vi "Was_string_matched.vi"(0 "Match Error":bool=TRUE, 1 "String Name":string, 2 "Variable name":string) -> ()   [LabVIEW 2010]
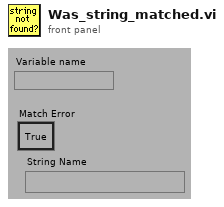
[diagram p1: front panel]
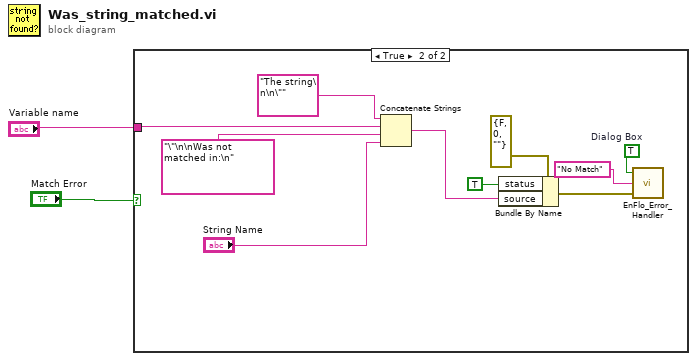
[diagram p0: block diagram]
diagram:
  n1 = case shown="True" "Match Error" {
    tunnel: "Variable name" -> [_ w10]
    frame False {
    }
    frame True {
      w7 = TRUE  # Dialog Box
      n2 = Concatenate Strings("The string\n\n\"", w10, "\"\n\nWas not matched in:\n", "String Name") -> (w5:string)
      n3 = Bundle By Name(cluster=errorcluster {"status"=FALSE, "code"=0, "source"=""} ("error in (no error)"), "status"=TRUE ("Bundle Element"), "source"=w5) -> (w8:errorcluster)
      n4 = call "EnFlo_Error_Handler.vi"("error in (no error)"=w8, "Error Type"="No Match", "Dialog Box (T)"=w7) -> ()  [unwired: 3 out]
    }
  }
